vi "Annotation_Read.vi"(7 "Unique labels":string[](array[string]), 8 "error in (no error)":errorcluster, 11 "Path":path) -> (0 "error out":errorcluster, 3 "Annotations (CWH)":T1[](array[typedef]) {"BBox"."x" format="%#_4p"; "BBox"."y" format="%#_4p"; "BBox"."w" format="%#_4p"; "BBox"."h" format="%#_4p"}, 5 "Class Names":string[](array[string]))   [LabVIEW 2020]
uses:
  <vilib>/Ngene/Deep Learning Toolkit/Toolkit/NN_Data/API/Data/Detection_Types/NN_BBox_Annotation.ctl
  <vilib>/Ngene/Deep Learning Toolkit/Toolkit/NN_Data/API/Data/Detection_Types/NN_BBox.ctl
  <vilib>/Utility/error.llb/whitespace.ctl
  <vilib>/Ngene/Deep Learning Toolkit/Toolkit/NN_Data/API/Data/Detection_Types/NN_BBox_Format_Conversion_Direction.ctl
  <vilib>/Ngene/Deep Learning Toolkit/Toolkit/Deep_Learning_Toolkit_by_Ngene.lvlib
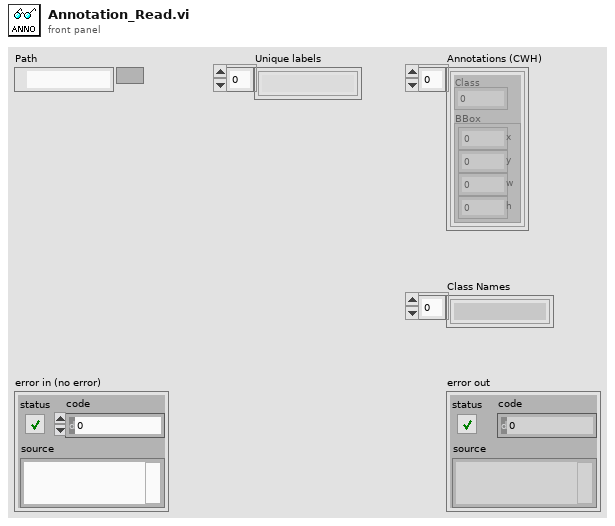
[diagram p1: front panel]
types:
  T1 = typedef "Deep_Learning_Toolkit_by_Ngene.lvlib/NN_BBox_Annotation.ctl" = cluster{"Class":i32, "BBox":T2}
  T2 = typedef "Deep_Learning_Toolkit_by_Ngene.lvlib/NN_BBox.ctl" = cluster{"x":sgl, "y":sgl, "w":sgl, "h":sgl}
  T3 = typedef "Deep_Learning_Toolkit_by_Ngene.lvlib/NN_BBox_Format_Conversion_Direction.ctl" = enum16{"SS_to_CWH", "CWH_to_SS"}
  T4 = typedef "whitespace.ctl" = u16
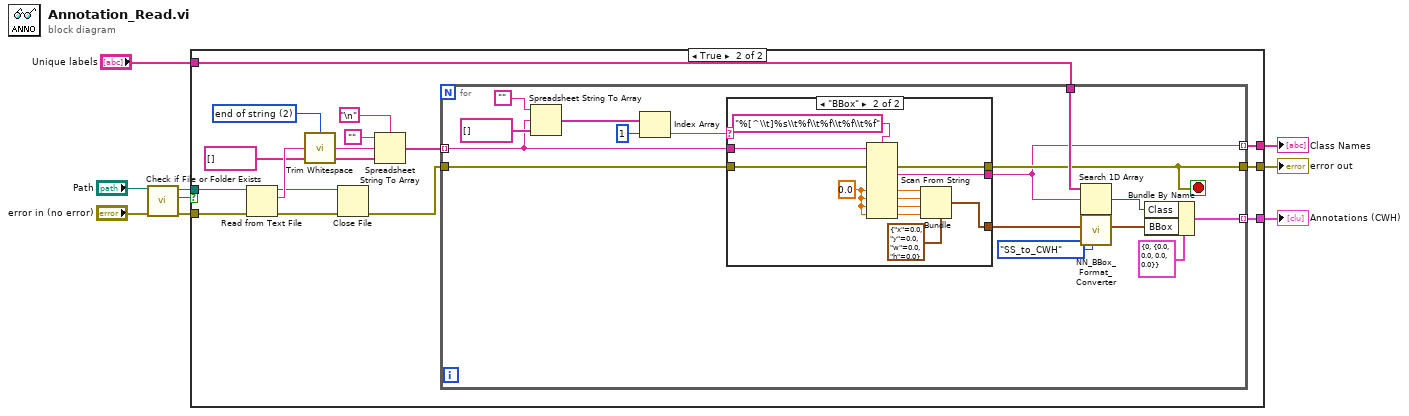
[diagram p0: block diagram]
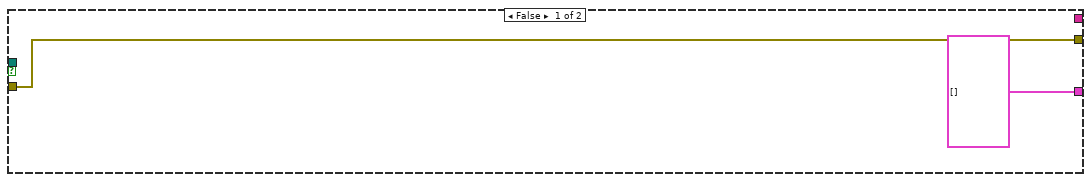
[diagram p2: hidden frame]
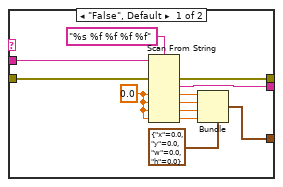
[diagram p3: hidden frame]
diagram:
  n1 = call <vilib>:"Check if File or Folder Exists.vi"("error in (no error)"="error in (no error)", "path"="Path") -> ("error out"=w4:errorcluster, "file or folder exists?"=w1:bool, "dup path"=w2:path)  [unwired: 7 in]
  n2 = case shown="True" w1 {
    tunnel: [w11 w26] -> w9
    tunnel: w2 -> [_ w25]
    tunnel: "Unique labels" -> [_ w24]
    tunnel: [T1[] [] w22] -> w7
    tunnel: w4 -> [w11 w17]
    tunnel: [_ w14] -> w5
    frame False {
    }
    frame True {
      w12 = T4 2 items=["both", "start of string", "end of string"] ("location (both)")
      n3 = Read from Text File(file (use dialog)=w25, error in=w17) -> (refnum out=w15:refnum<file>, text=w23:string, error out=w16:errorcluster)  [unwired: 2 in, 1 out]
      n4 = call <vilib>:"Trim Whitespace.vi"("string"=w23, "location (both)"=w12) -> ("trimmed string"=w13:string)
      n5 = Close File(refnum=w15, error in=w16) -> (error out=w27:errorcluster)  [unwired: 1 out]
      n6 = Spreadsheet String To Array(delimiter (Tab)="\n", format string="", spreadsheet string=w13, array type (2D Dbl)=string[] []) -> (array=w20:string[])
      n7 = for {
        tunnel: w20 -> [w30] mode=indexing
        tunnel: w27 -> [w39]
        tunnel: [w32] -> w26
        tunnel: w24 -> [w38]
        tunnel: [w33] -> w22 mode=indexing
        tunnel: [w29] -> w14 mode=indexing
        stop <- w32 stop-if-true
        n8 = Spreadsheet String To Array(format string="", spreadsheet string=w30, array type (2D Dbl)=string[] []) -> (array=w42:string[])  [unwired: 1 in]
        n9 = Index Array(array=w42, index=1) -> (element=w40:string)
        n10 = case shown="\"BBox\"" w40 {
          tunnel: w30 -> [w54 w67]
          tunnel: w39 -> [w53 w66]
          tunnel: [w52 w65] -> w32
          tunnel: [w45 w57] -> w35
          tunnel: [w44 w58] -> w29
          frame "False", Default {
            w49 = sgl 0.0 ("h")
            n11 = Scan From String(format string="%s %f %f %f %f", input string=w54, error in=w53, default 2=w49, default 3=w49, default 4=w49, default 5=w49) -> (error out=w52:errorcluster, output 1=w44:string, output 2=w50:sgl, output 3=w48:sgl, output 4=w47:sgl, output 5=w46:sgl)  [unwired: 2 in, 2 out]
            n12 = Bundle(cluster=T2 {"x"=0.0, "y"=0.0, "w"=0.0, "h"=0.0} ("Box"), "x"=w50, "y"=w48, "w"=w47, "h"=w46) -> (w45:T2)
          }
          frame "BBox" {
            w59 = sgl 0.0 ("h")
            n13 = Scan From String(format string="%[^\\t]%s\\t%f\\t%f\\t%f\\t%f", input string=w67, error in=w66, default 3=w59, default 4=w59, default 5=w59, default 6=w59) -> (error out=w65:errorcluster, output 1=w58:string, output 3=w63:sgl, output 4=w62:sgl, output 5=w61:sgl, output 6=w60:sgl)  [unwired: 4 in, 2 out]
            n14 = Bundle(cluster=T2 {"x"=0.0, "y"=0.0, "w"=0.0, "h"=0.0} ("Box"), "x"=w63, "y"=w62, "w"=w61, "h"=w60) -> (w57:T2)
          }
        }
        n15 = Search 1D Array(1D array=w38, element=w29) -> (index of element=w37:i32)  [unwired: 1 in]
        n16 = call <vilib>:"NN_BBox_Format_Converter.vi"("Conversion_Direction"=NN_BBox_Format_Conversion_Direction."SS_to_CWH" ("Format_Transform"), "BBox in"=w35) -> ("BBox out"=w28:T2)  [unwired: 9 in]
        n17 = Bundle By Name(cluster=T1 {"Class"=0, "BBox"={"x"=0.0, "y"=0.0, "w"=0.0, "h"=0.0}} ("BoxC"), "Class"=w37, "BBox"=w28) -> (w33:T1)
      }
    }
  }
  "error out" <- w9
  "Annotations (CWH)" <- w7
  "Class Names" <- w5
